vi "fit orbit from queues.vi"(0 "magnetometer set queue":refnum<queue>, 1 "timeout in ms (-1)":i32=20, 2 "display queues":T5, 5 "error in (no error)":errorcluster, 6 "reinitialize fitter":bool, 8 "accumulate fixed parameters":bool, 9 "reset fixed parameters?":bool) -> (14 "orbit parameters":T4, 15 "new fit":bool, 16 "orbit for display":T3 {"height above sensor" format="%.1f"; "y offset" format="%.1f"; "x offset" format="%.1f"; "magnet tilt (deg)" format="%.1f"; "axis angle (deg)" format="%.1f"; "minor axis" format="%.1f"; "maj axis" format="%.1f"}, 17 "intrinsic parameters":T1, 19 "error out":errorcluster)   [LabVIEW 2017]
uses:
  typedefs/queue cluster.ctl
  typedefs/reading queue.ctl
  typedefs/reading.ctl
  typedefs/readingType.ctl
  typedefs/magnetomter reading set.ctl
  typedefs/orbit parameters with crossing info.ctl
  typedefs/magnet location with timestamp.ctl
  <vilib>/Utility/error.llb/Clear Errors.vi
  popup panels/control panel globals.vi
panel:
  out "XY Graph":T2(graph)
  out "time to fit":u32
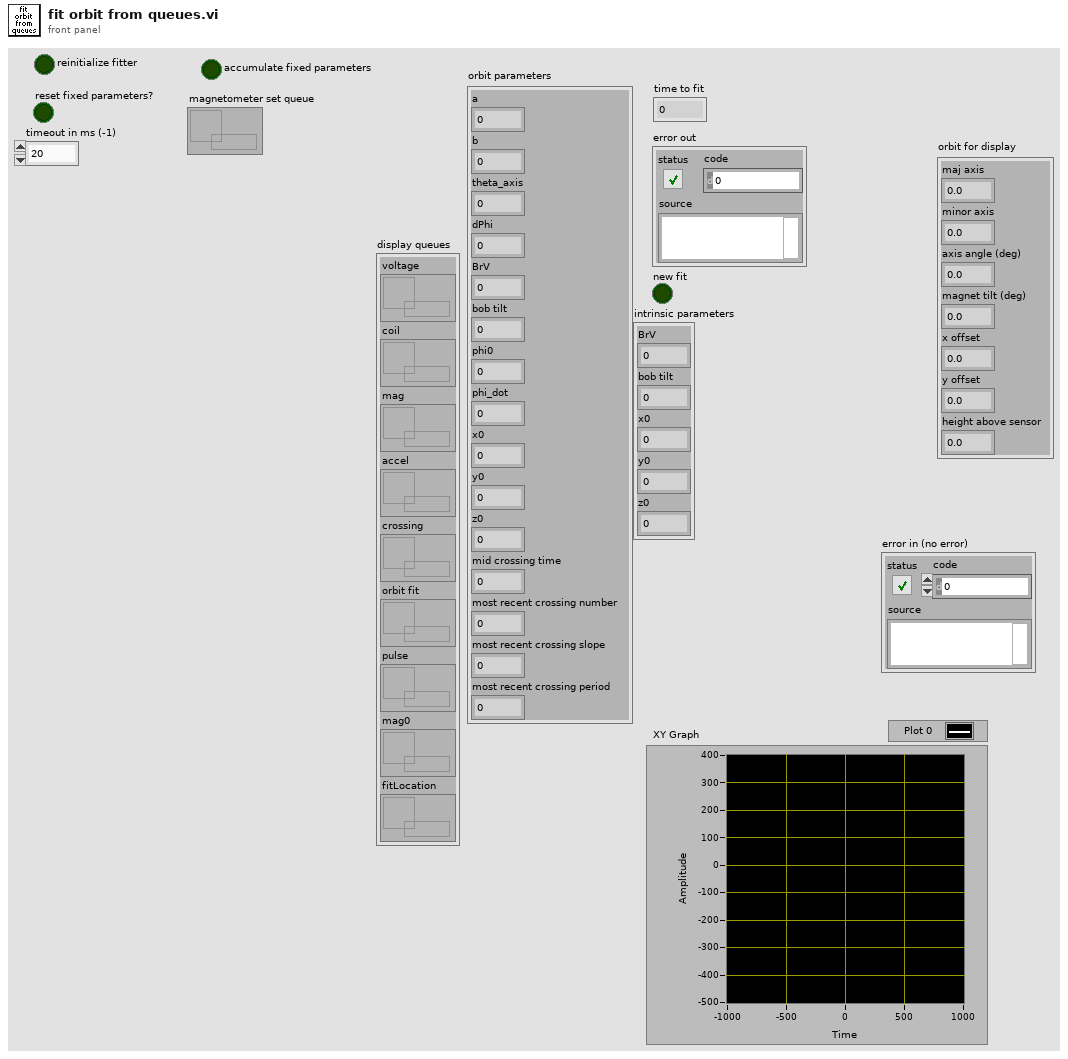
[diagram p1: front panel]
types:
  T1 = cluster{"BrV":dbl, "bob tilt":dbl, "x0":dbl, "y0":dbl, "z0":dbl}
  T2 = cluster{"sensor0 measured":dbl[], "sensor0 measured":dbl[]}[]
  T3 = cluster{"maj axis":dbl, "minor axis":dbl, "axis angle (deg)":dbl, "magnet tilt (deg)":dbl, "x offset":dbl, "y offset":dbl, "height above sensor":dbl}
  T4 = typedef "orbit parameters with crossing info.ctl" = cluster{"a":dbl, "b":dbl, "theta_axis":dbl, "dPhi":dbl, "BrV":dbl, "bob tilt":dbl, "phi0":dbl, "phi_dot":dbl, "x0":dbl, "y0":dbl, "z0":dbl, "mid crossing time":dbl, "most recent crossing number":dbl, "most recent crossing slope":dbl, "most recent crossing period":dbl}
  T5 = typedef "queue cluster.ctl" = cluster{"voltage":T6, "coil":T6, "mag":refnum<queue>, "accel":T6, "crossing":T6, "orbit fit":refnum<queue>, "pulse":T6, "mag0":T6, "fitLocation":refnum<queue>}
  T6 = typedef "reading queue.ctl" = refnum<queue>
  T7 = typedef "crossing stats.ctl" = cluster{"recent crossing":dbl, "prev crossing":dbl, "crossing-2":dbl, "number of crossings":i32, "period":dbl, "new crossing":bool, "new odd crossing":bool, "slope":dbl}
  T8 = typedef "orbit parameters full.ctl" = cluster{"a":dbl, "b":dbl, "theta_axis":dbl, "dPhi":dbl, "BrV":dbl, "bob tilt":dbl, "phi0":dbl, "phi_dot":dbl, "x0":dbl, "y0":dbl, "z0":dbl}
  T9 = typedef "magnetomter reading set.ctl" = cluster{"time":fxp<+,48,48>, "mag readings":cluster{"magnetometer index":dbl, "Bx":dbl, "By":dbl, "Bz":dbl, "magnetometer x":dbl, "magnetometer y":dbl}[]}
  T10 = cluster{"a":dbl, "b":dbl, "theta_axis":dbl, "bob tilt":dbl, "x0":dbl, "y0":dbl, "z0":dbl}
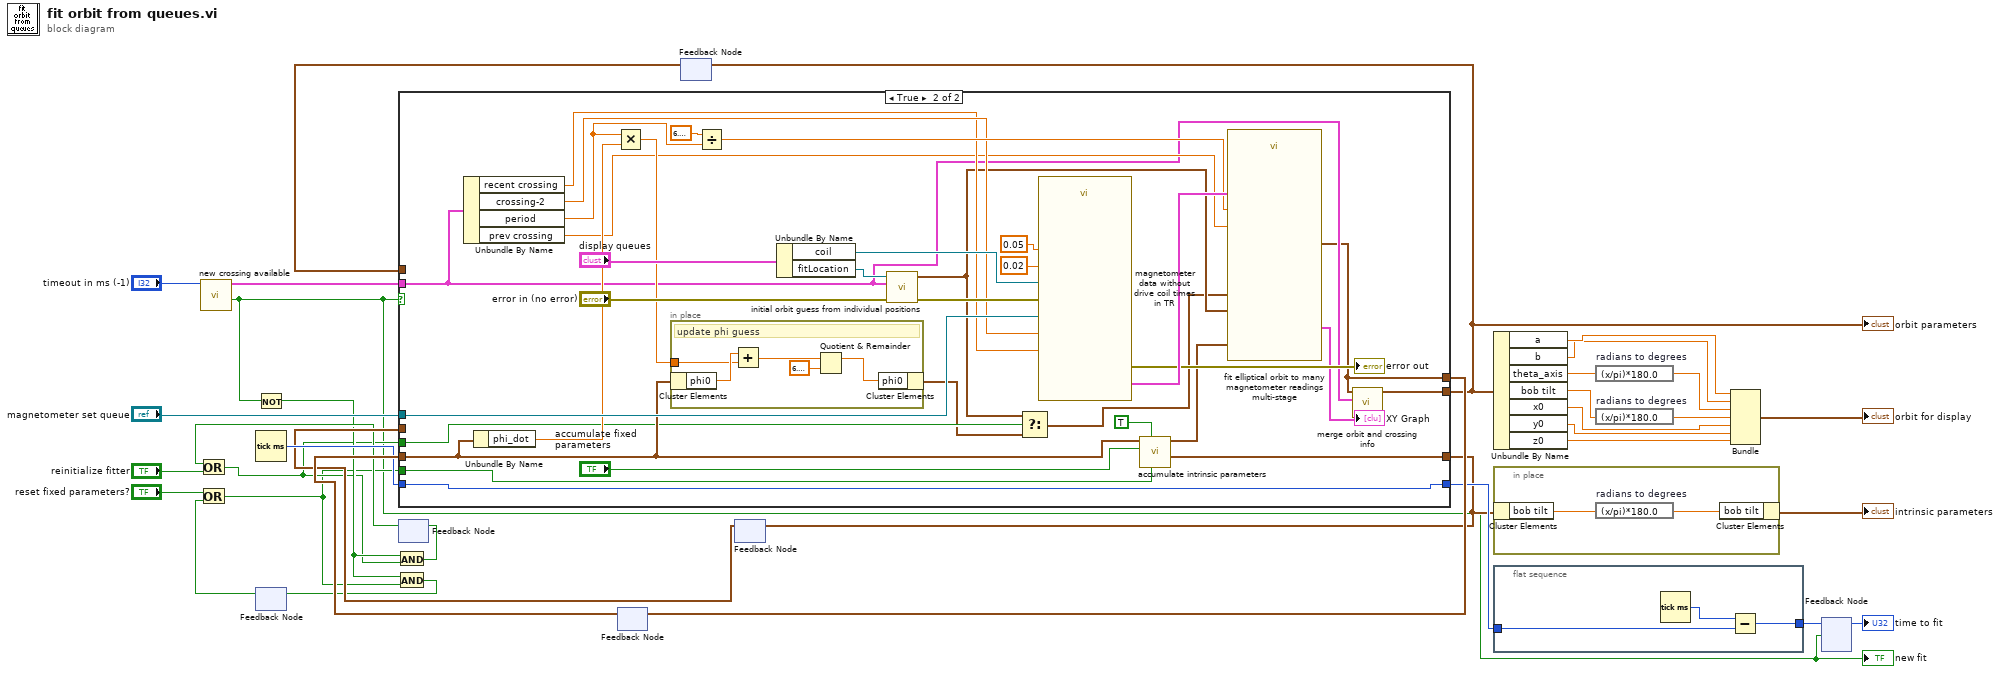
[diagram p0: block diagram]
diagram:
  n1 = call "new crossing available.vi"("timeout in ms (-1)"="timeout in ms (-1)") -> ("new odd crossing"=w3:bool, "crossing stats"=w2:T7)  [unwired: 7 in, 2 out]
  "new fit" <- w3
  n2 = Not(x=w3) -> (.not. x?=w9:bool)
  n3 = Tick Count (ms)() -> (millisecond timer value=w31:u32)
  n4 = feedback #1() -> (w8:bool)  [unwired: 1 in]
  n5 = Or(x="reset fixed parameters?", y=w8) -> (x .or. y?=w4:bool)
  n6 = And(x=w9, y=w4) -> (x .and. y?=w6:bool)
  n7 = feedback-in #1(w6) -> ()
  n8 = feedback #2() -> (w11:bool)  [unwired: 1 in]
  n9 = Or(x=w11, y="reinitialize fitter") -> (x .or. y?=w5:bool)
  n10 = And(x=w9, y=w5) -> (x .and. y?=w10:bool)
  n11 = feedback-in #2(w10) -> ()
  n12 = feedback #3() -> (w32:T8)  [unwired: 1 in]
  n13 = feedback #4() -> (w27:T4)  [unwired: 1 in]
  n14 = feedback #5() -> (w15:T1)  [unwired: 1 in]
  n15 = case shown="True" w3 {
    tunnel: "magnetometer set queue" -> [_ w66]
    tunnel: w2 -> [_ w51]
    tunnel: [w37 w50] -> w33
    tunnel: w32 -> [w37 w47]
    tunnel: w31 -> [_ w53]
    tunnel: [_ w53] -> w30
    tunnel: [w36 w49] -> w26
    tunnel: w27 -> [w36 _]
    tunnel: [w35 w44] -> w14
    tunnel: w15 -> [w35 _]
    tunnel: w5 -> [_ w42]
    tunnel: w4 -> [_ w38]
    frame False {
    }
    frame True {
      n16 = Unbundle By Name(w51) -> ("recent crossing"=w57:dbl, "crossing-2"=w59:dbl, "period"=w56:dbl, "prev crossing"=w52:dbl)
      n17 = Unbundle By Name(w47) -> ("phi_dot"=w55:dbl)
      n18 = Multiply(x=w56, y=w55) -> (x*y=w54:dbl)
      n19 = in-place {
        in-place-border: w54 -> [w74]
        # "update phi guess"
        n20 = in-place-cluster #6(w47) -> ("phi0"=w75:dbl)
        n21 = Add(x=w75, y=w74) -> (x+y=w73:dbl)
        n22 = Quotient & Remainder(x=w73, y=6.283185307179586) -> (x-y*floor(x/y)=w72:dbl)  [unwired: 1 out]
        n23 = in-place-cluster #6("phi0"=w72) -> (w41:T8)
      }
      n24 = Divide(x=6.283185307179586, y=w56) -> (x/y=w60:dbl)
      n25 = Unbundle By Name("display queues") -> ("coil"=w69:T6, "fitLocation"=w65:refnum<queue>)
      n26 = call "initial orbit guess from individual positions.vi"("error in (no error)"="error in (no error)", "crossing stats"=w51, "fitLocation queue"=w65) -> ("error out"=w64:errorcluster, "initial guess"=w40:T8)  [unwired: 7 in]
      n27 = Select(t=w40, s=w42, f=w41) -> (s? t:f=w39:T8)
      n28 = call "magnetometer data without drive coil times in TR.vi"("magnetometer set queue"=w66, "buffer (s) after"=0.05, "t1"=w57, "coil"=w69, "error in (no error)"=w64, "buffer (s) before"=0.02, "t0"=w59) -> ("mag readings no coil"=w62:T9[], "error out"=→"error out":errorcluster)  [unwired: 7 in]
      n29 = call "accumulate intrinsic parameters.vi"("reset fixed parameters?"=w38, "use fixed parameters?"=TRUE, "accumulate fixed parameters"="accumulate fixed parameters", "fit parameters"=w47) -> ("intrinsic parameters"=w44:T1, "fixed parameter input to ftter"=w46:T8)  [unwired: 6 in]
      n30 = call "fit elliptical orbit to many magnetometer readings multi-stage.vi"("initial parameters 1"=w39, "fixed parameters"=w46, "initial parameters 2"=w40, "magnetometer readings"=w62, "omega"=w60, "t0"=w52) -> ("fit parameters"=w50:T8, "fit graph"=→"XY Graph":T2)  [unwired: 5 in, 3 out]
      n31 = call "merge orbit and crossing info.vi"("crossing stats"=w51, "orbit parameters"=w50) -> ("orbit parameters with crossing"=w49:T4)  [unwired: 9 in]
    }
  }
  "orbit parameters" <- w26
  n32 = feedback-in #3(w33) -> ()
  n33 = feedback-in #4(w26) -> ()
  n34 = feedback-in #5(w14) -> ()
  n35 = Unbundle By Name(w26) -> ("a"=w23:dbl, "b"=w22:dbl, "theta_axis"=w25:dbl, "bob tilt"=w24:dbl, "x0"=w19:dbl, "y0"=w18:dbl, "z0"=w17:dbl)
  n36 = in-place {
    n37 = in-place-cluster #7(w14) -> ("bob tilt"=w77:dbl)
    n38 = expression code="(x/pi)*180.0" "radians to degrees"(w77) -> (w76:dbl)
    n39 = in-place-cluster #7("bob tilt"=w76) -> (→"intrinsic parameters":T1)
  }
  n40 = flat-sequence {
    tunnel: w30 -> [w79]
    tunnel: [w78] -> w29
    frame #0 {
      n41 = Tick Count (ms)() -> (millisecond timer value=w80:u32)
      n42 = Subtract(x=w80, y=w79) -> (x-y=w78:u32)
    }
  }
  n43 = expression code="(x/pi)*180.0" "radians to degrees"(w25) -> (w21:dbl)
  n44 = expression code="(x/pi)*180.0" "radians to degrees"(w24) -> (w20:dbl)
  n45 = Bundle("a"=w23, "b"=w22, "theta_axis"=w21, "bob tilt"=w20, "x0"=w19, "y0"=w18, "z0"=w17) -> (→"orbit for display":T10)  [unwired: 1 in]
  n46 = feedback-in #8(w29, w3) -> ()
  n47 = feedback #8() -> (→"time to fit":u32)  [unwired: 1 in]
